vi "Handle Error (User).vi"(8 "error in":errorcluster, 11 "Node in":refnum<class "ThermotronDriver.lvclass">) -> (0 "error out":errorcluster, 3 "Node out":refnum<class "ThermotronDriver.lvclass">)   [LabVIEW 2023, in "ThermotronDriver.lvlib" / "ThermotronDriver.lvclass"]
uses:
  ThermotronDriver.lvclass
  ThermotronDriver.lvclass/ThermotronDriver.ctl
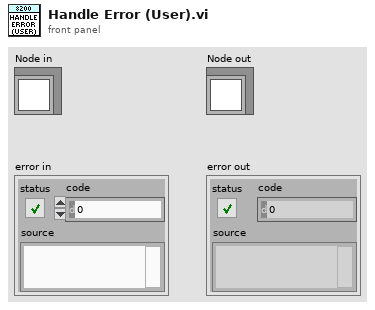
[diagram p1: front panel]
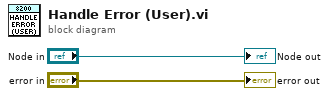
[diagram p0: block diagram]
diagram:
  "error out" <- "error in"
  "Node out" <- "Node in"
